vi "Initiate Synchronous Generation.vi"(0 "instrument handle":refnum<k15>, 5 "Synchronization Configuration":T1={"RF Delay Range (s)"=2e-06, "RF Delay (s)"=0.0} {"RF Delay (s)" format="%#_6p"; "RF Delay Range (s)" format="%#_6p"}, 11 "error in (no error)":errorcluster) -> (4 "instrument handle out":refnum<k15>, 15 "error out":errorcluster)   [LabVIEW 2016, in "Envelope Tracking.lvlib"]
uses:
  Envelope Tracking.lvlib
  Typedefs/Synchronization Configuration.ctl
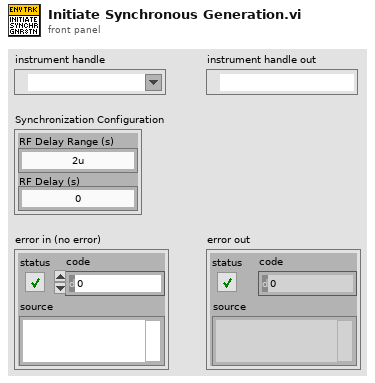
[diagram p1: front panel]
types:
  T1 = typedef "Envelope Tracking.lvlib/Synchronization Configuration.ctl" = cluster{"RF Delay Range (s)":sgl, "RF Delay (s)":sgl}
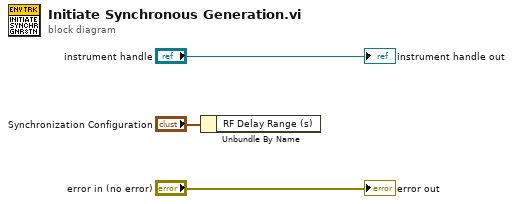
[diagram p0: block diagram]
diagram:
  n1 = Unbundle By Name("Synchronization Configuration") -> ()  [unwired: 1 out]
  "instrument handle out" <- "instrument handle"
  "error out" <- "error in (no error)"
